vi "Práctica7.1_DAQ0804.vi"() -> ()   [LabVIEW 2018]
panel:
  in  "Alto":bool
  out "Entrada analógica":dbl(knob) scale=0.0..5.0
  in  "Entrada analógica":dbl(knob) scale=0.0..5.0
  out "Entradas digitales":bool[](array[boolean])
  in  "Salidas digitales":bool[](array[boolean])
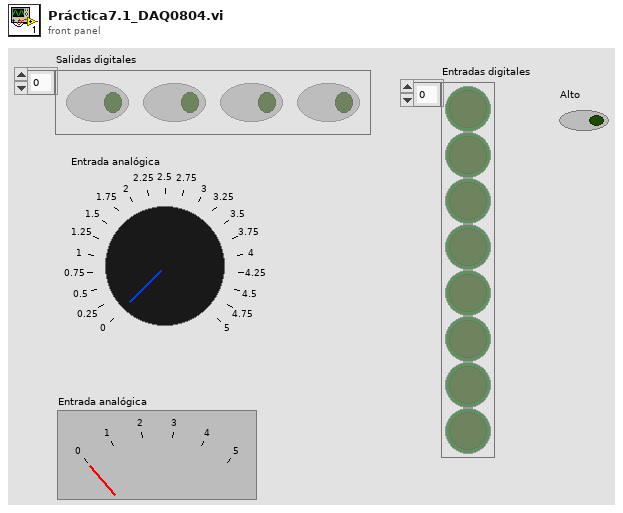
[diagram p1: front panel]
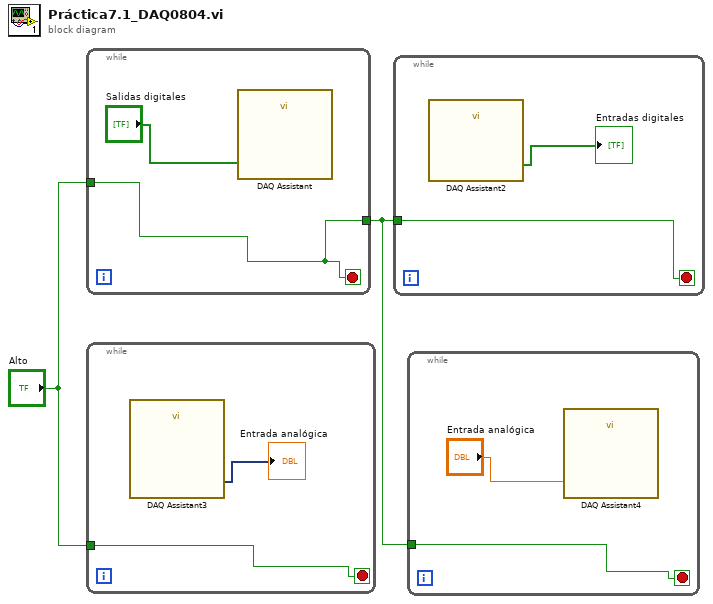
[diagram p0: block diagram]
diagram:
  n1 = while {
    tunnel: "Alto" -> [w4]
    tunnel: [w4] -> w1
    stop <- w4 stop-if-true
    n2 = call "DAQ Assistant"("data"="Salidas digitales") -> ()  [unwired: 17 in, 2 out]
  }
  n3 = while {
    tunnel: "Alto" -> [w5]
    stop <- w5 stop-if-true
    n4 = call "DAQ Assistant3"() -> ("data"=→"Entrada analógica":dynamicdata)  [unwired: 17 in, 2 out]
  }
  n5 = while {
    tunnel: w1 -> [w8]
    stop <- w8 stop-if-true
    n6 = call "DAQ Assistant2"() -> ("data"=→"Entradas digitales":bool[])  [unwired: 17 in, 2 out]
  }
  n7 = while {
    tunnel: w1 -> [w10]
    stop <- w10 stop-if-true
    n8 = call "DAQ Assistant4"("data"="Entrada analógica") -> ()  [unwired: 17 in, 2 out]
  }
